vi "GetAsyncErrors.vi"(8 "error in (no error)":errorcluster, 9 "timeout in ms (-1)":i32=-1, 11 "YActor in":refnum<class "YActor.lvclass">) -> (0 "error out":errorcluster, 3 "YActor out":refnum<class "YActor.lvclass">)   [LabVIEW 2021, in "YActor.lvclass"]
doc: "Author: Patriek Bruins\nCompany: Philips\nDepartment: PInS TMA\n\nCopyright © 2017\nAll rights reserved. This VI or any portion thereof may not be used in any application created outside of the Royal Philips company without the express written permission of the author."
uses:
  YActor.lvclass
  YActor.lvclass/YActor.ctl
panel:
  # "Author: Patriek Bruins\nCompany: Philips\nDepartment: PInS TMA\n\nCopyright © 2017\nAll rights reserved. This VI or any portion thereof may not be used in any application created outside of the Royal Philips company without the express written permission of the author."
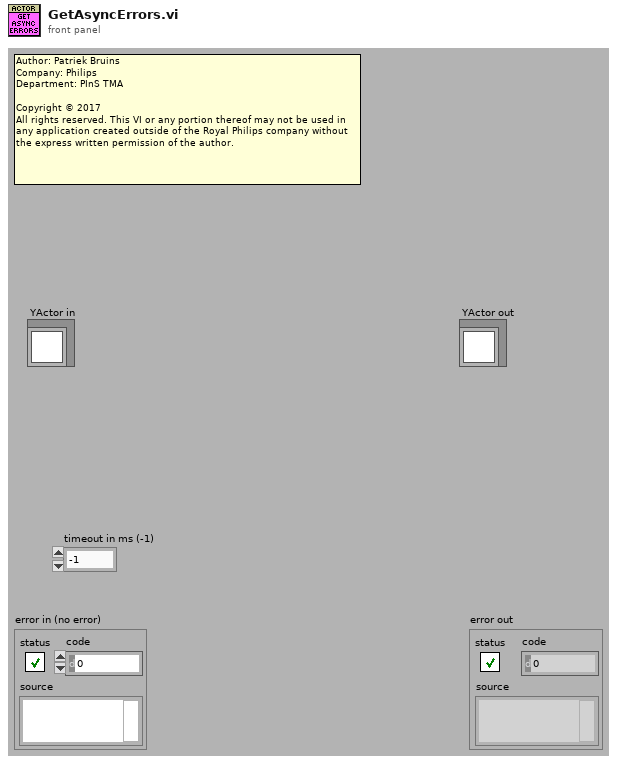
[diagram p1: front panel]
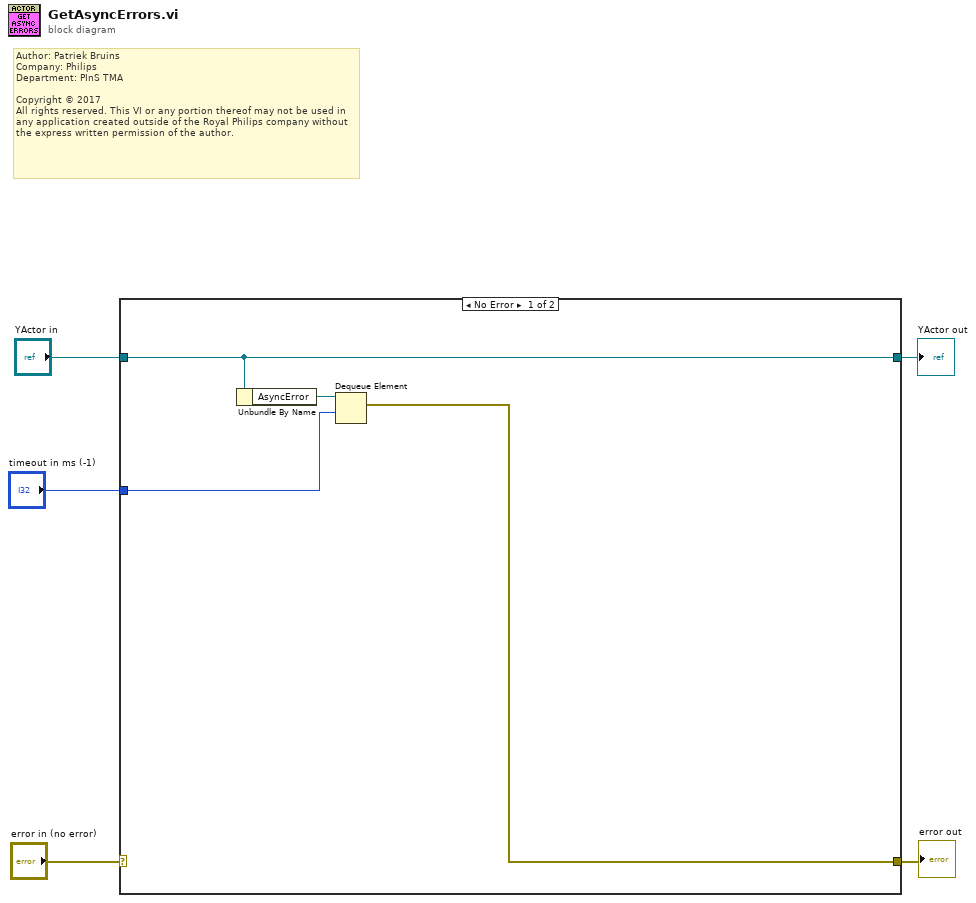
[diagram p0: block diagram]
diagram:
  # "Author: Patriek Bruins\nCompany: Philips\nDepartment: PInS TMA\n\nCopyright © 2017\nAll rights reserved. This VI or any portion thereof may not be used in any application created outside of the Royal Philips company without the express written permission of the author."
  n1 = case shown="No Error" "error in (no error)" {
    selector: "error in (no error)" -> [_ w11]
    tunnel: [w7 w11] -> w4
    tunnel: [w9 w10] -> w2
    tunnel: "YActor in" -> [w9 w10]
    tunnel: "timeout in ms (-1)" -> [w6 _]
    frame No Error {
      n2 = Unbundle By Name(w9) -> ("AsyncError"=w8:refnum<queue>)
      n3 = Dequeue Element(queue=w8, timeout in ms (-1)=w6) -> (element=w7:errorcluster)  [unwired: 1 in, 3 out]
    }
    frame Error {
    }
  }
  "error out" <- w4
  "YActor out" <- w2
